vi "test ClearData.vi"(8 "error in (no error)":errorcluster, 11 "TestCase in":refnum<class "Data Manipulation Tests.lvclass">) -> (0 "error out":errorcluster, 3 "TestCase out":refnum<class "Data Manipulation Tests.lvclass">)   [LabVIEW 2017, in "Pointer Tests.lvlib" / "Data Manipulation Tests.lvclass"]
uses:
  Data Manipulation Tests.lvclass
  Source/Classes/Pointer/Public/New/New (1B).vi
  Source/Classes/Pointer/Public/Write/Write (1D U8).vi
  Source/Classes/Pointer/Public/Read/Read (1D U8).vi
  <vilib>/addons/_JKI Toolkits/VI Tester/TestCase.llb/TestCase.lvclass
  Source/Classes/Pointer/Pointer.lvclass
  C:/Program Files (x86)/National Instruments/LabVIEW 2017/vi.lib/addons/_JKI Toolkits/VI Tester/TestCase.llb/TestCase.lvclass
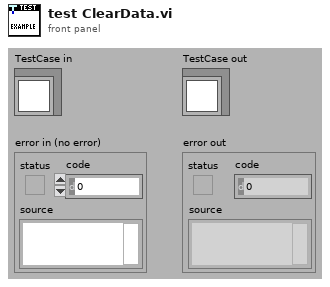
[diagram p1: front panel]
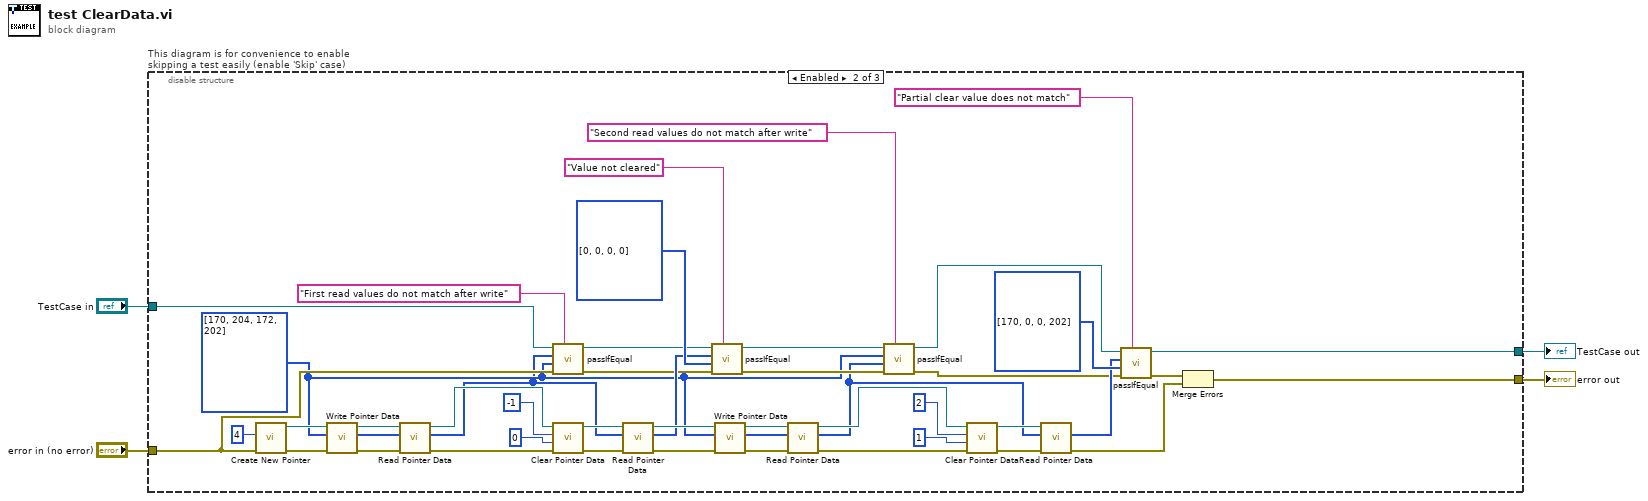
[diagram p0: block diagram]
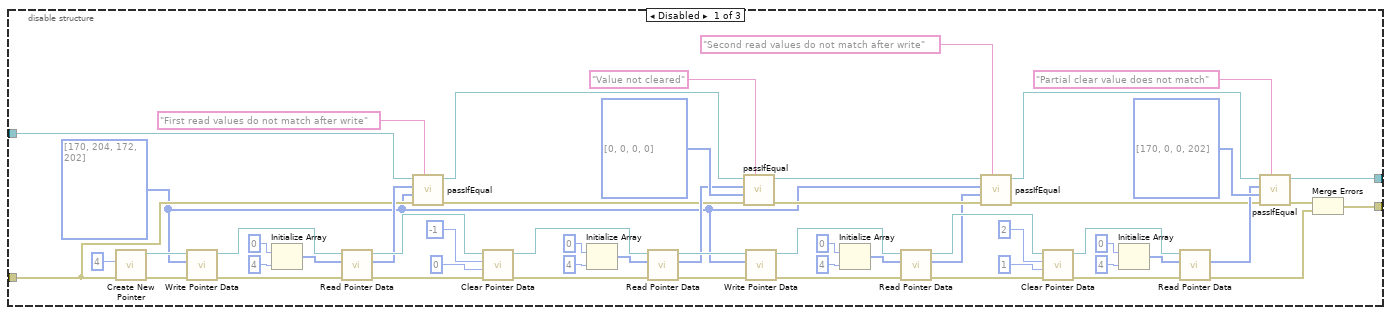
[diagram p2: hidden frame]
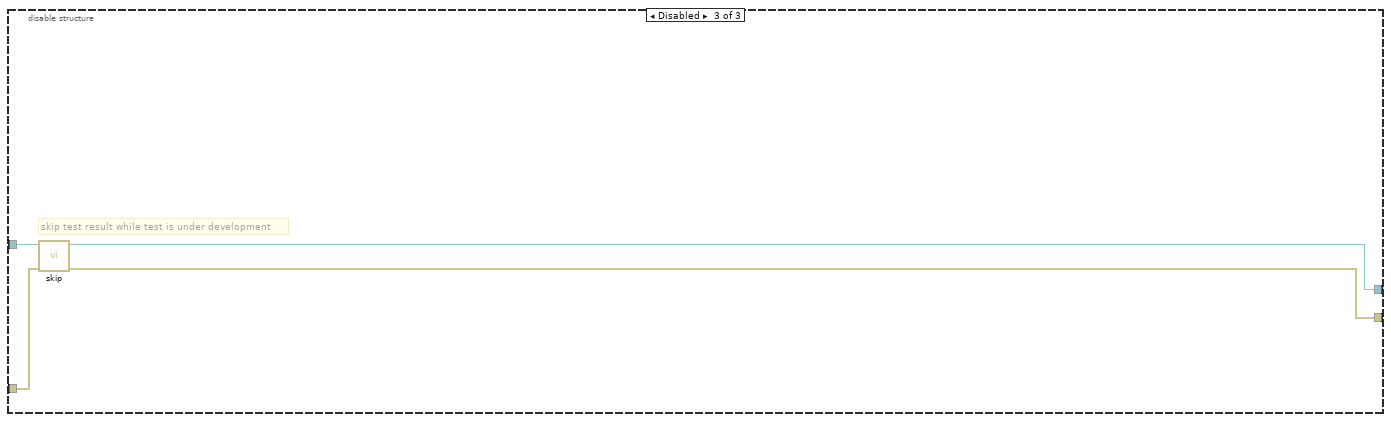
[diagram p3: hidden frame]
diagram:
  n1 = disable-structure "This diagram is for convenience to enable skipping a test easily (enable 'Skip' case)" shown="Enabled" {
    disable-tunnel: "TestCase in" -> [w33 w79 w110]
    disable-tunnel: [w51 w97 w108] -> w1
    disable-tunnel: [w48 w94 w109] -> w3
    disable-tunnel: "error in (no error)" -> [w30 w77 w107]
    frame Disabled {
      w17 = u8[] [170, 204, 172, 202] ("buffer in")
      n2 = call-poly "Create New Pointer.vi"("error in (no error)"=w30, "count (1)"=u64 4) -> ("error out"=w50:errorcluster, "Pointer"=w60:refnum<class "Pointer.lvclass">)  [unwired: 8 in]
      n3 = call-poly "Write Pointer Data.vi"("error in (no error)"=w50, "buffer in"=w17, "Pointer in"=w60) -> ("error out"=w46:errorcluster, "Pointer out"=w35:refnum<class "Pointer.lvclass">)  [unwired: 5 in, 2 out]
      n4 = Initialize Array(u8 0 ("value"), 4 ("dimension size")) -> (w14:u8[])
      n5 = call-poly "Read Pointer Data.vi"("error in (no error)"=w46, "buffer in"=w14, "Pointer in"=w35) -> ("error out"=w36:errorcluster, "buffer out"=w31:u8[], "Pointer out"=w34:refnum<class "Pointer.lvclass">)  [unwired: 5 in, 1 out]
      n6 = call-dynamic "passIfEqual.vi"("custom report message (\"\")"="First read values do not match after write" ("custom report message (\"\")"), "error in (no error)"=w30, "y"=w17, "x"=w31, "TestCase in"=w33) -> ("error out"=w29:errorcluster, "TestCase out"=w32:refnum<class "Data Manipulation Tests.lvclass">)  [unwired: 5 in]
      n7 = call "Clear Pointer Data.vi"("error in (no error)"=w36, "offset (0)"=u64 0, "length (-1: rest)"=i64 -1, "Pointer in"=w34) -> ("error out"=w45:errorcluster, "Pointer out"=w44:refnum<class "Pointer.lvclass">)  [unwired: 6 in]
      n8 = Initialize Array(u8 0 ("value"), 4 ("dimension size")) -> (w11:u8[])
      n9 = call-poly "Read Pointer Data.vi"("error in (no error)"=w45, "buffer in"=w11, "Pointer in"=w44) -> ("error out"=w49:errorcluster, "buffer out"=w43:u8[], "Pointer out"=w58:refnum<class "Pointer.lvclass">)  [unwired: 5 in, 1 out]
      n10 = call-dynamic "passIfEqual.vi"("custom report message (\"\")"="Value not cleared" ("custom report message (\"\")"), "error in (no error)"=w29, "y"=u8[] [0, 0, 0, 0] ("buffer in"), "x"=w43, "TestCase in"=w32) -> ("error out"=w53:errorcluster, "TestCase out"=w24:refnum<class "Data Manipulation Tests.lvclass">)  [unwired: 5 in]
      n11 = call-poly "Write Pointer Data.vi"("error in (no error)"=w49, "buffer in"=w17, "Pointer in"=w58) -> ("error out"=w57:errorcluster, "Pointer out"=w27:refnum<class "Pointer.lvclass">)  [unwired: 5 in, 2 out]
      n12 = Initialize Array(u8 0 ("value"), 4 ("dimension size")) -> (w8:u8[])
      n13 = call-poly "Read Pointer Data.vi"("error in (no error)"=w57, "buffer in"=w8, "Pointer in"=w27) -> ("error out"=w28:errorcluster, "buffer out"=w22:u8[], "Pointer out"=w26:refnum<class "Pointer.lvclass">)  [unwired: 5 in, 1 out]
      n14 = call-dynamic "passIfEqual.vi"("custom report message (\"\")"="Second read values do not match after write" ("custom report message (\"\")"), "error in (no error)"=w53, "y"=w22, "x"=w17, "TestCase in"=w24) -> ("error out"=w25:errorcluster, "TestCase out"=w23:refnum<class "Data Manipulation Tests.lvclass">)  [unwired: 5 in]
      n15 = call "Clear Pointer Data.vi"("error in (no error)"=w28, "offset (0)"=u64 1, "length (-1: rest)"=i64 2, "Pointer in"=w26) -> ("error out"=w42:errorcluster, "Pointer out"=w41:refnum<class "Pointer.lvclass">)  [unwired: 6 in]
      n16 = Initialize Array(u8 0 ("value"), 4 ("dimension size")) -> (w5:u8[])
      n17 = call-poly "Read Pointer Data.vi"("error in (no error)"=w42, "buffer in"=w5, "Pointer in"=w41) -> ("error out"=w47:errorcluster, "buffer out"=w54:u8[])  [unwired: 5 in, 2 out]
      n18 = call-dynamic "passIfEqual.vi"("custom report message (\"\")"="Partial clear value does not match" ("custom report message (\"\")"), "error in (no error)"=w25, "y"=u8[] [170, 0, 0, 202] ("buffer in"), "x"=w54, "TestCase in"=w23) -> ("error out"=w52:errorcluster, "TestCase out"=w51:refnum<class "Data Manipulation Tests.lvclass">)  [unwired: 5 in]
      n19 = Merge Errors(w52, w47) -> (w48:errorcluster)
    }
    frame Enabled {
      w65 = u8[] [170, 204, 172, 202] ("buffer in")
      n20 = call-poly "Create New Pointer.vi"("error in (no error)"=w77, "count (1)"=u64 4) -> ("error out"=w96:errorcluster, "Pointer"=w106:refnum<class "Pointer.lvclass">)  [unwired: 8 in]
      n21 = call-poly "Write Pointer Data.vi"("error in (no error)"=w96, "buffer in"=w65, "Pointer in"=w106) -> ("error out"=w92:errorcluster, "buffer out"=w64:u8[], "Pointer out"=w81:refnum<class "Pointer.lvclass">)  [unwired: 5 in, 1 out]
      n22 = call-poly "Read Pointer Data.vi"("error in (no error)"=w92, "buffer in"=w64, "Pointer in"=w81) -> ("error out"=w82:errorcluster, "buffer out"=w63:u8[], "Pointer out"=w80:refnum<class "Pointer.lvclass">)  [unwired: 5 in, 1 out]
      n23 = call-dynamic "passIfEqual.vi"("custom report message (\"\")"="First read values do not match after write" ("custom report message (\"\")"), "error in (no error)"=w77, "y"=w65, "x"=w63, "TestCase in"=w79) -> ("error out"=w76:errorcluster, "TestCase out"=w78:refnum<class "Data Manipulation Tests.lvclass">)  [unwired: 5 in]
      n24 = call "Clear Pointer Data.vi"("error in (no error)"=w82, "offset (0)"=u64 0, "length (-1: rest)"=i64 -1, "Pointer in"=w80) -> ("error out"=w91:errorcluster, "Pointer out"=w90:refnum<class "Pointer.lvclass">)  [unwired: 6 in]
      n25 = call-poly "Read Pointer Data.vi"("error in (no error)"=w91, "buffer in"=w63, "Pointer in"=w90) -> ("error out"=w95:errorcluster, "buffer out"=w89:u8[], "Pointer out"=w104:refnum<class "Pointer.lvclass">)  [unwired: 5 in, 1 out]
      n26 = call-dynamic "passIfEqual.vi"("custom report message (\"\")"="Value not cleared" ("custom report message (\"\")"), "error in (no error)"=w76, "y"=u8[] [0, 0, 0, 0] ("buffer in"), "x"=w89, "TestCase in"=w78) -> ("error out"=w99:errorcluster, "TestCase out"=w71:refnum<class "Data Manipulation Tests.lvclass">)  [unwired: 5 in]
      n27 = call-poly "Write Pointer Data.vi"("error in (no error)"=w95, "buffer in"=w65, "Pointer in"=w104) -> ("error out"=w103:errorcluster, "buffer out"=w62:u8[], "Pointer out"=w74:refnum<class "Pointer.lvclass">)  [unwired: 5 in, 1 out]
      n28 = call-poly "Read Pointer Data.vi"("error in (no error)"=w103, "buffer in"=w62, "Pointer in"=w74) -> ("error out"=w75:errorcluster, "buffer out"=w61:u8[], "Pointer out"=w73:refnum<class "Pointer.lvclass">)  [unwired: 5 in, 1 out]
      n29 = call-dynamic "passIfEqual.vi"("custom report message (\"\")"="Second read values do not match after write" ("custom report message (\"\")"), "error in (no error)"=w99, "y"=w61, "x"=w65, "TestCase in"=w71) -> ("error out"=w72:errorcluster, "TestCase out"=w70:refnum<class "Data Manipulation Tests.lvclass">)  [unwired: 5 in]
      n30 = call "Clear Pointer Data.vi"("error in (no error)"=w75, "offset (0)"=u64 1, "length (-1: rest)"=i64 2, "Pointer in"=w73) -> ("error out"=w88:errorcluster, "Pointer out"=w87:refnum<class "Pointer.lvclass">)  [unwired: 6 in]
      n31 = call-poly "Read Pointer Data.vi"("error in (no error)"=w88, "buffer in"=w61, "Pointer in"=w87) -> ("error out"=w93:errorcluster, "buffer out"=w100:u8[])  [unwired: 5 in, 2 out]
      n32 = call-dynamic "passIfEqual.vi"("custom report message (\"\")"="Partial clear value does not match" ("custom report message (\"\")"), "error in (no error)"=w72, "y"=u8[] [170, 0, 0, 202] ("buffer in"), "x"=w100, "TestCase in"=w70) -> ("error out"=w98:errorcluster, "TestCase out"=w97:refnum<class "Data Manipulation Tests.lvclass">)  [unwired: 5 in]
      n33 = Merge Errors(w98, w93) -> (w94:errorcluster)
    }
    frame Disabled {
      # "skip test result while test is under development"
      n34 = call <vilib>:"skip.vi"("error in (no error)"=w107, "TestCase in"=w110) -> ("error out"=w109:errorcluster, "TestCase out"=w108:refnum<class "Data Manipulation Tests.lvclass">)  [unwired: 8 in]
    }
  }
  "error out" <- w3
  "TestCase out" <- w1
